vi "Get XML Item Name.vi"(8 "error in":errorcluster, 11 "Node":refnum<k20>) -> (0 "error out":errorcluster, 2 "Name":string, 3 "Node out":refnum<k20>)   [LabVIEW 2020, in "Template Tool.lvlib"]
uses:
  Template Tool.lvlib
  <resource>/objmgr/DOMUserDefRef.rc
  <vilib>/xml/NI_XML.lvlib
  <vilib>/xml/Close Reference(NNMap).vi
  <vilib>/xml/Close Reference(Node).vi
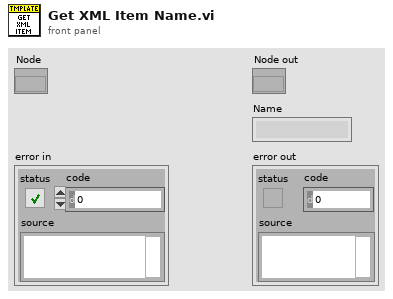
[diagram p1: front panel]
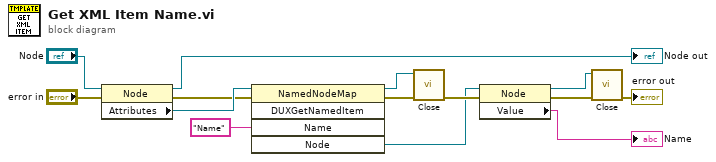
[diagram p0: block diagram]
diagram:
  n1 = property class="Node"(reference="Node", error in="error in") -> (reference out=→"Node out":refnum<k20>, error out=w12:errorcluster, "Attributes"=w13:refnum<k20>)
  n2 = invoke class="NamedNodeMap" method="DUXGetNamedItem"(reference=w13, error in=w12, "Name"="Name") -> (reference out=w9:refnum<k20>, error out=w11:errorcluster, "Node"=w8:refnum<k20>)  [unwired: 2 in, 2 out]
  n3 = call-poly <vilib>:"Close.vi"("error in (no error)"=w11, "named node map"=w9) -> ("error out"=w10:errorcluster)  [unwired: 7 in]
  n4 = property class="Node"(reference=w8, error in=w10) -> (reference out=w6:refnum<k20>, error out=w7:errorcluster, "Value"=→"Name":string)
  n5 = call-poly <vilib>:"Close.vi"("error in (no error)"=w7, "node"=w6) -> ("error out"=→"error out":errorcluster)  [unwired: 7 in]
